vi "Static Read.vi"(8 "error in (no error)":errorcluster, 11 "Abs_Time in":refnum<class "Abs_Variant 1D.lvclass">) -> (0 "error out":errorcluster, 2 "Value":T1, 3 "Abs_Time out":refnum<class "Abs_Variant 1D.lvclass">)   [LabVIEW 2021, in "Abs_Variant 1D.lvclass"]
uses:
  Abs_Variant 1D.lvclass
  Support/Type.ctl
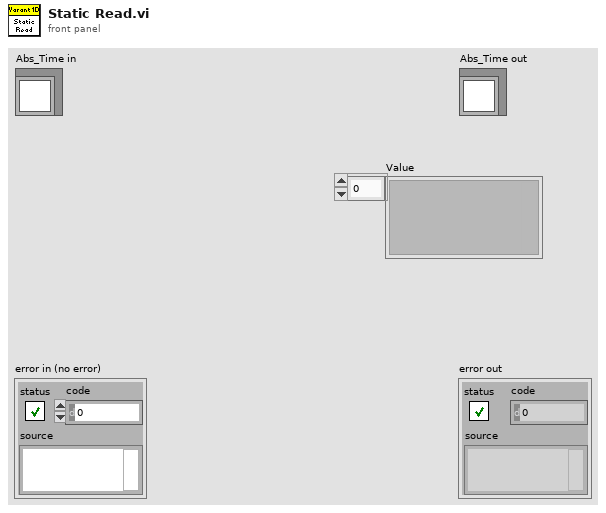
[diagram p1: front panel]
types:
  T1 = typedef "Abs_Variant 1D.lvclass/Type.ctl" = variant[]
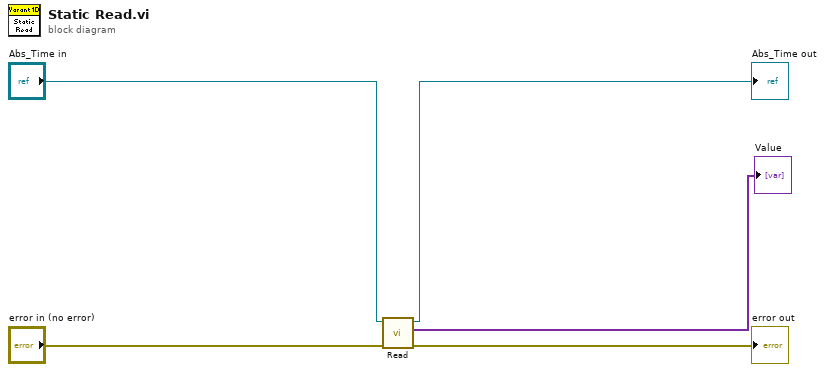
[diagram p0: block diagram]
diagram:
  n1 = call-dynamic "Read.vi"("error in (no error)"="error in (no error)", "Double Float.lvclass_340760 in"="Abs_Time in") -> ("error out"=→"error out":errorcluster, "Value"=→"Value":T1, "Double Float.lvclass_340760 out"=→"Abs_Time out":refnum<class "Abs_Variant 1D.lvclass">)  [unwired: 7 in]
